vi "Dashboard_Operations.vi"   [LabVIEW 2020]
uses:
  <vilib>/Rock Robotics/Network Tables/NT Read Number.vi
  Systems/Shooter/Determiner/Shooter_Globals.vi
  Globals/Feeder_Globals.vi
  <vilib>/Rock Robotics/Network Tables/NT Read Boolean.vi
  Globals/Drive_Globals.vi
  Globals/Turret_Globals.vi
  <vilib>/Rock Robotics/Network Tables/NT Write Boolean.vi
  Globals/Flywheel_Globals.vi
  Globals/Sensor_Values.vi
  <vilib>/Rock Robotics/Network Tables/NT Write Number.vi
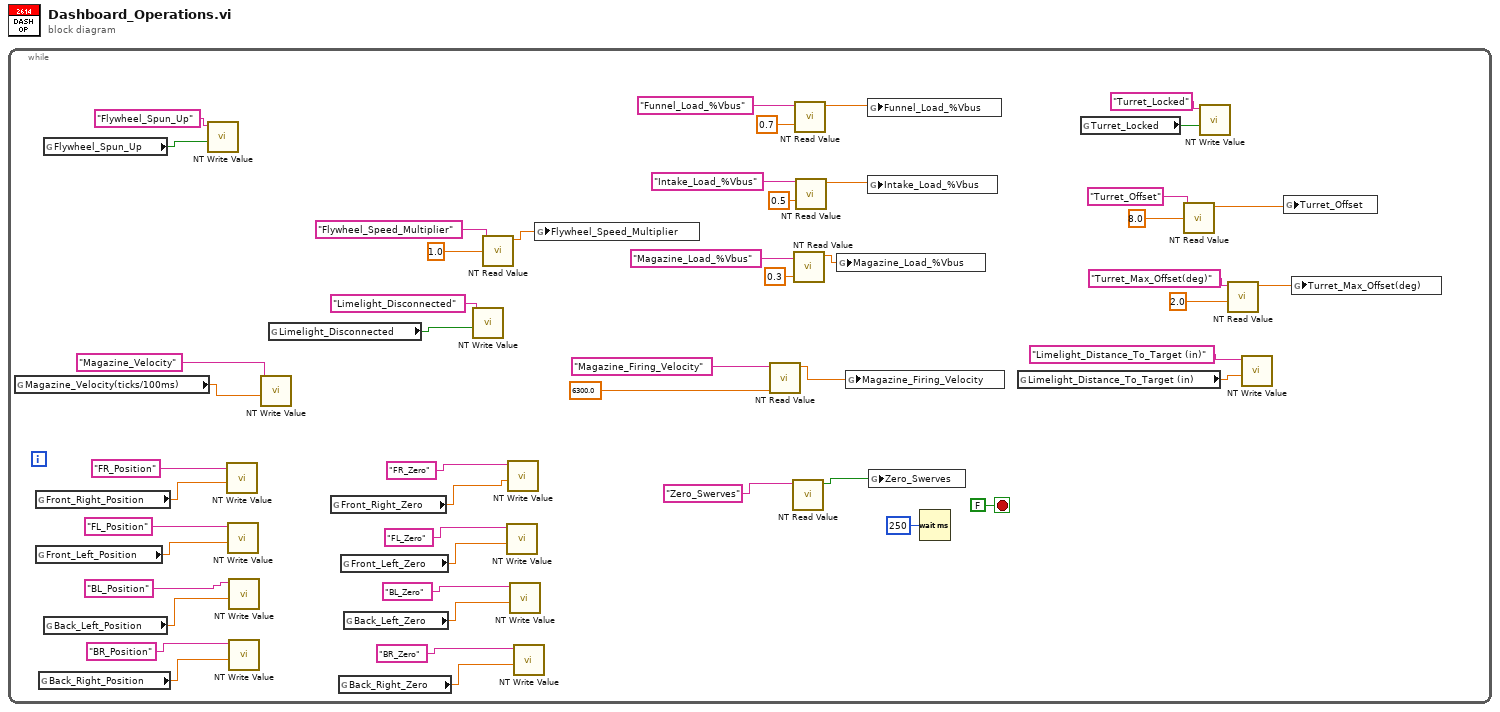
[diagram p0: block diagram]
diagram:
  n1 = while {
    stop <- FALSE stop-if-true
    n2 = global read "Sensor_Values.vi" "Magazine_Velocity(ticks/100ms)"() -> (w33:dbl)
    n3 = global read "Drive_Globals.vi" "Front_Right_Position"() -> (w20:dbl)
    n4 = global read "Drive_Globals.vi" "Front_Left_Position"() -> (w29:dbl)
    n5 = global read "Drive_Globals.vi" "Back_Right_Position"() -> (w16:dbl)
    n6 = global read "Flywheel_Globals.vi" "Flywheel_Spun_Up"() -> (w45:bool)
    n7 = global read "Drive_Globals.vi" "Back_Left_Position"() -> (w27:dbl)
    n8 = call-poly <vilib>:"NT Write Value.vi"("Boolean"=w45, "Name"="Flywheel_Spun_Up") -> ()  [unwired: 9 in, 1 out]
    n9 = call-poly <vilib>:"NT Write Value.vi"("Numeric"=w20, "Name"="FR_Position") -> ()  [unwired: 9 in, 1 out]
    n10 = call-poly <vilib>:"NT Write Value.vi"("Numeric"=w29, "Name"="FL_Position") -> ()  [unwired: 9 in, 1 out]
    n11 = call-poly <vilib>:"NT Write Value.vi"("Numeric"=w27, "Name"="BL_Position") -> ()  [unwired: 9 in, 1 out]
    n12 = call-poly <vilib>:"NT Write Value.vi"("Numeric"=w16, "Name"="BR_Position") -> ()  [unwired: 9 in, 1 out]
    n13 = call-poly <vilib>:"NT Write Value.vi"("Numeric"=w33, "Name"="Magazine_Velocity") -> ()  [unwired: 9 in, 1 out]
    n14 = global read "Sensor_Values.vi" "Limelight_Disconnected"() -> (w13:bool)
    n15 = global read "Drive_Globals.vi" "Front_Right_Zero"() -> (w25:dbl)
    n16 = global read "Drive_Globals.vi" "Back_Right_Zero"() -> (w15:dbl)
    n17 = global read "Drive_Globals.vi" "Front_Left_Zero"() -> (w23:dbl)
    n18 = global read "Drive_Globals.vi" "Back_Left_Zero"() -> (w19:dbl)
    n19 = call-poly <vilib>:"NT Write Value.vi"("Boolean"=w13, "Name"="Limelight_Disconnected") -> ()  [unwired: 9 in, 1 out]
    n20 = call-poly <vilib>:"NT Read Value.vi"("Default Value"=1.0, "Name"="Flywheel_Speed_Multiplier") -> ("Numeric"=w37:dbl)  [unwired: 8 in, 1 out]
    n21 = call-poly <vilib>:"NT Write Value.vi"("Numeric"=w23, "Name"="FL_Zero") -> ()  [unwired: 9 in, 1 out]
    n22 = call-poly <vilib>:"NT Write Value.vi"("Numeric"=w25, "Name"="FR_Zero") -> ()  [unwired: 9 in, 1 out]
    n23 = call-poly <vilib>:"NT Write Value.vi"("Numeric"=w19, "Name"="BL_Zero") -> ()  [unwired: 9 in, 1 out]
    n24 = call-poly <vilib>:"NT Write Value.vi"("Numeric"=w15, "Name"="BR_Zero") -> ()  [unwired: 9 in, 1 out]
    n25 = global write "Shooter_Globals.vi" "Flywheel_Speed_Multiplier"(w37) -> ()
    n26 = call-poly <vilib>:"NT Read Value.vi"("Default Value"=6300.0, "Name"="Magazine_Firing_Velocity") -> ("Numeric"=w35:dbl)  [unwired: 8 in, 1 out]
    n27 = call-poly <vilib>:"NT Read Value.vi"("Name"="Zero_Swerves") -> ("Boolean"=w31:bool)  [unwired: 9 in, 1 out]
    n28 = call-poly <vilib>:"NT Read Value.vi"("Default Value"=0.3, "Name"="Magazine_Load_%Vbus") -> ("Numeric"=w41:dbl)  [unwired: 8 in, 1 out]
    n29 = call-poly <vilib>:"NT Read Value.vi"("Default Value"=0.7, "Name"="Funnel_Load_%Vbus") -> ("Numeric"=w49:dbl)  [unwired: 8 in, 1 out]
    n30 = call-poly <vilib>:"NT Read Value.vi"("Default Value"=0.5, "Name"="Intake_Load_%Vbus") -> ("Numeric"=w47:dbl)  [unwired: 8 in, 1 out]
    n31 = global write "Feeder_Globals.vi" "Magazine_Load_%Vbus"(w41) -> ()
    n32 = global write "Feeder_Globals.vi" "Magazine_Firing_Velocity"(w35) -> ()
    n33 = global write "Feeder_Globals.vi" "Funnel_Load_%Vbus"(w49) -> ()
    n34 = global write "Feeder_Globals.vi" "Intake_Load_%Vbus"(w47) -> ()
    n35 = global write "Drive_Globals.vi" "Zero_Swerves"(w31) -> ()
    n36 = Wait (ms)(milliseconds to wait=u32 250) -> ()  [unwired: 1 out]
    n37 = global read "Sensor_Values.vi" "Limelight_Distance_To_Target (in)"() -> (w3:dbl)
    n38 = global read "Turret_Globals.vi" "Turret_Locked"() -> (w51:bool)
    n39 = call-poly <vilib>:"NT Read Value.vi"("Default Value"=8.0, "Name"="Turret_Offset") -> ("Numeric"=w9:dbl)  [unwired: 8 in, 1 out]
    n40 = call-poly <vilib>:"NT Write Value.vi"("Boolean"=w51, "Name"="Turret_Locked") -> ()  [unwired: 9 in, 1 out]
    n41 = call-poly <vilib>:"NT Read Value.vi"("Default Value"=2.0, "Name"="Turret_Max_Offset(deg)") -> ("Numeric"=w2:dbl)  [unwired: 8 in, 1 out]
    n42 = call-poly <vilib>:"NT Write Value.vi"("Numeric"=w3, "Name"="Limelight_Distance_To_Target (in)") -> ()  [unwired: 9 in, 1 out]
    n43 = global write "Turret_Globals.vi" "Turret_Offset"(w9) -> ()
    n44 = global write "Turret_Globals.vi" "Turret_Max_Offset(deg)"(w2) -> ()
  }
